vi "status_flag_names.vi"() -> (2 "Names":string[](array[string]))   [LabVIEW 2013]
uses:
  status_flag.ctl
panel:
  out "Flag dummy":T1
  # "Return an array of strings naming the status flags.\nAs of LV 2010 SP1, there were some interactions with\nthe execution properties for what we do here to work\n(getting a property from the control)  In particular, \nit seems that this VI can't be reentrant."
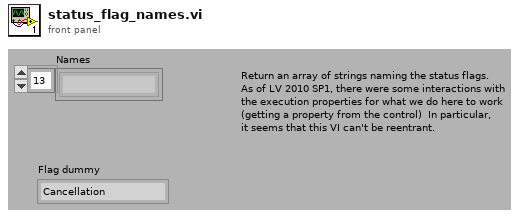
[diagram p1: front panel]
types:
  T1 = typedef "status_flag.ctl" = enum16{"Cancellation", "Goal filter", "Valid position", "Goal saturation tip", "Goal saturation RCM", "Goal circle saturation", "Position saturation", "Output saturation", "Acceleration limiting", "Finished late", "Stimulus increasing", "Integral error saturation", "Velocity limiting", "Log warning", "Log error", "Link KF degraded"}
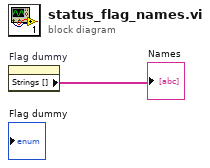
[diagram p0: block diagram]
diagram:
  n1 = property on="Flag dummy" class="Enum (strict)"() -> ("Strings []"=→"Names":string[])  [unwired: 2 in, 2 out]
